vi "Set References.vi"(6 "Test Information":refnum<vi>, 8 "error in (no error)":errorcluster, 9 "Status References":refnum<vi>[](array[refnum]), 10 "Serial References":refnum<vi>[](array[refnum]), 11 "Acrobat Template in":refnum<class "Application.lvclass">) -> (0 "error out":errorcluster, 3 "Acrobat Template out":refnum<class "Application.lvclass">)   [LabVIEW 2017, in "Application.lvlib" / "Application.lvclass"]
uses:
  Application.lvclass
  typedefs/Test Info -- Cluster.ctl
  Application.lvclass/Application.ctl
  Properties/App Properties.lvclass
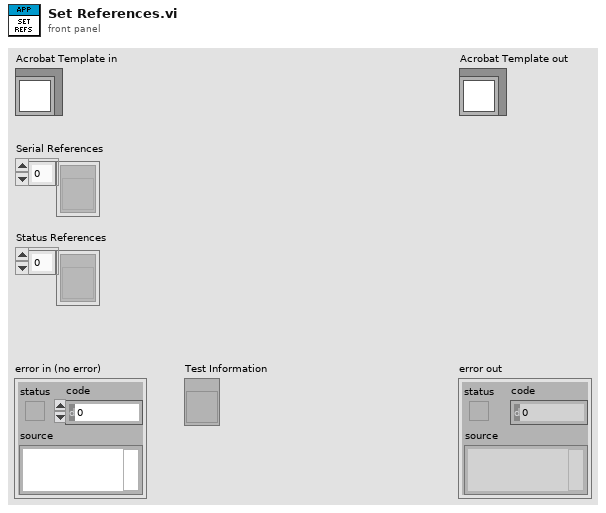
[diagram p1: front panel]
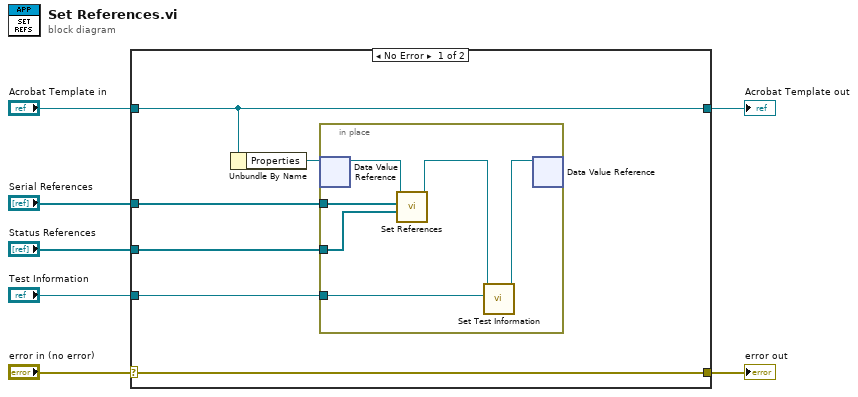
[diagram p0: block diagram]
diagram:
  n1 = case shown="No Error" "error in (no error)" {
    selector: "error in (no error)" -> [w13 w21]
    tunnel: [w13 w21] -> w6
    tunnel: [w12 w20] -> w4
    tunnel: "Acrobat Template in" -> [w12 w20]
    tunnel: "Serial References" -> [w10 _]
    tunnel: "Status References" -> [w9 _]
    tunnel: "Test Information" -> [w8 _]
    frame No Error {
      n2 = Unbundle By Name(w12) -> ("Properties"=w11:refnum<data-value>)
      n3 = in-place {
        in-place-border: w10 -> [w15]
        in-place-border: w9 -> [w14]
        in-place-border: w8 -> [w19]
        n4 = in-place-dvr #1(w11) -> (w17:refnum<class "App Properties.lvclass">)  [unwired: 1 out]
        n5 = call-dynamic "Set References.vi"("Status References"=w14, "Serial References"=w15, "Template Properties in"=w17) -> ("Template Properties out"=w16:refnum<class "App Properties.lvclass">)  [unwired: 7 in, 1 out]
        n6 = call-dynamic "Set Test Information.vi"("Test Information"=w19, "Template Properties in"=w16) -> ("Template Properties out"=w18:refnum<class "App Properties.lvclass">)  [unwired: 8 in, 1 out]
        n7 = in-place-dvr #1(w18) -> ()  [unwired: 2 out]
      }
    }
    frame Error {
    }
  }
  "error out" <- w6
  "Acrobat Template out" <- w4
